vi "backup pagecount.vi"(8 "error in (no error)":errorcluster, 11 "backup_ref":u64) -> (0 "error out":errorcluster)   [LabVIEW 2020, in "sqlite3.lvlib"]
uses:
  sqlite3.lvlib
  bin/sqlite3_64.dll
panel:
  out "pagecount":i32
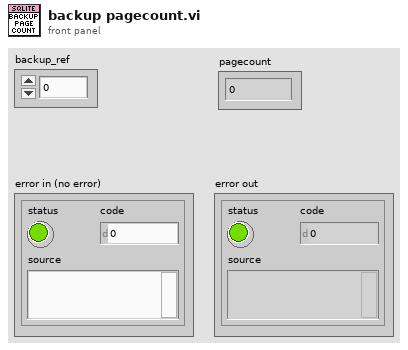
[diagram p1: front panel]
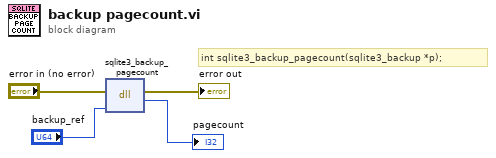
[diagram p0: block diagram]
diagram:
  # "int sqlite3_backup_pagecount(sqlite3_backup *p);"
  n1 = dll-call lib="D:/Project/Labview-Projects/database-configuration/externals/sqlite3/Source/bin/sqlite3_*.*" fn="sqlite3_backup_pagecount"(error in="error in (no error)", "backup_ref"="backup_ref") -> (error out=→"error out":errorcluster, "return type"=→"pagecount":i32)  [unwired: 3 in, 1 out]
